vi "Close TDMS.vi"(8 "error in (no error)":errorcluster, 11 "Honeywell Compass HMC6343":refnum<class "Honeywell Compass HMC6343.lvclass">) -> (0 "error out":errorcluster, 3 "Honeywell Compass HMC6343 out":refnum<class "Honeywell Compass HMC6343.lvclass">)   [LabVIEW 2019, in "Honeywell Compass HMC6343.lvclass"]
doc: "Closes the TDMS file."
uses:
  Honeywell Compass HMC6343.lvclass
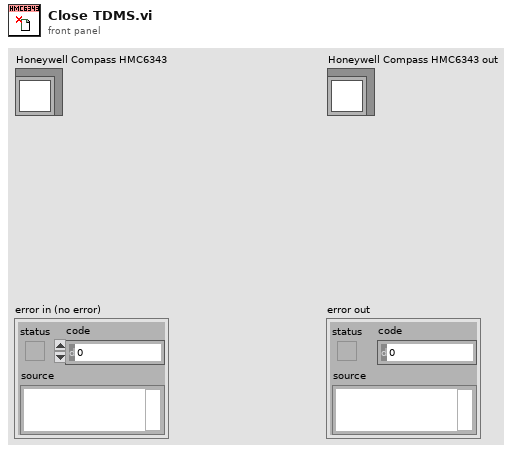
[diagram p1: front panel]
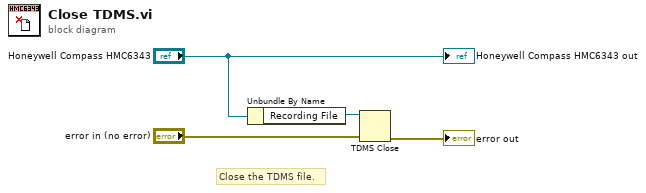
[diagram p0: block diagram]
diagram:
  # "Close the TDMS file."
  n1 = Unbundle By Name("Honeywell Compass HMC6343") -> ("Recording File"=w3:refnum<k34>)
  n2 = TDMS Close(8:"error in (no error)", 11:w3) -> (0:→"error out":errorcluster)  [unwired: 1 out]
  "Honeywell Compass HMC6343 out" <- "Honeywell Compass HMC6343"
